vi "Test Executive.vi"(11 "Module Config":T30={"Name"="Test Executive", "Parent Q"=refnum, "Is Child?"=FALSE, "Index"=0, "Dirs"={"Root"=path "C:/MTE", "Config"=path "C:/MTE/Config", "Logs"=path "C:/MTE/Logs", "Reports"=path "C:/ATE/Reports", "App Data"=path "C:/ProgramData/Test Executive"}, "Simulate"=FALSE, "SimCtrl"=refnum}) -> ()   [LabVIEW 2018] (continued)
          frame "Simulate OFF", "Simulate ON" {
            n2666 = call <vilib>:"Menu.Simulate, Set Menu State.vi"("Menu Tag"=w5387, "Menu Ref"=w5388) -> ("Sim ON"=w5386:bool)  [unwired: 8 in, 1 out]
            n2667 = To Variant(anything=w5386) -> (Variant=w5390:variant)
            n2668 = call <vilib>:"Q.Enqueue App.vi"("Data1"=w5390, "Task Name"="Simulate", "Q In"=w5391) -> ()  [unwired: 7 in, 2 out]
          }
          frame "Show Station Module" {
            n2669 = call <vilib>:"Q.Enqueue Task.vi"("Task Name"="Station Module - Show", "Q In"=w5393) -> ()  [unwired: 8 in, 2 out]
          }
          frame "Mode Manager" {
            n2670 = call <vilib>:"Q.Enqueue Task.vi"("Task Name"="Config - Mode Manager", "Q In"=w5395) -> ()  [unwired: 8 in, 2 out]
          }
          frame "Local Station" {
            n2671 = call <vilib>:"Q.Enqueue Task.vi"("Task Name"="Config - Set Local Station Cfg", "Q In"=w5397) -> ()  [unwired: 8 in, 2 out]
          }
          frame "Test Executive" {
            n2672 = call <vilib>:"Q.Enqueue Task.vi"("Task Name"="Config - Set Test Exec Cfg", "Q In"=w5399) -> ()  [unwired: 8 in, 2 out]
          }
          frame "File Sync" {
            n2673 = To Variant(anything=TRUE) -> (Variant=w5400:variant)
            n2674 = call <vilib>:"Q.Enqueue Task.vi"("Data1"=w5400, "Task Name"="Config - Set File Sync", "Q In"=w5403) -> ()  [unwired: 7 in, 2 out]
          }
          frame "File Rotate" {
            n2675 = call <vilib>:"File.Rotate.Manager - Config Dialog.vi"("QName"="FileRotate") -> ()  [unwired: 9 in, 2 out]
          }
          frame "Test Reports" {
            n2676 = To Variant(anything=TRUE) -> (Variant=w5405:variant)
            n2677 = call <vilib>:"Q.Enqueue Task.vi"("Data1"=w5405, "Task Name"="Config - Set Reports", "Q In"=w5408) -> ()  [unwired: 7 in, 2 out]
          }
          frame "Route Check" {
            n2678 = call <vilib>:"Q.Enqueue Task.vi"("Task Name"="Route Check", "Q In"=w5410) -> ()  [unwired: 8 in, 2 out]
          }
          frame "Show PLC State" {
            n2679 = call <vilib>:"Q.Enqueue Task.vi"("Task Name"="PLC - Show State", "Q In"=w5412) -> ()  [unwired: 8 in, 2 out]
          }
          frame "Show Block Diagram" {
            n2680 = call <vilib>:"Module.Window, Q Task.vi"("Action"=Window.Task,_Action."Open Block Diagram()", "Q In"=w5414) -> ()  [unwired: 8 in, 2 out]
          }
          frame "Go to Maint Tab" {
            n2681 = call <vilib>:"Module.Window, Q Task.vi"("Show"=TRUE, "Action"=Window.Task,_Action."Go To Maint Tab()", "Q In"=w5417) -> ()  [unwired: 7 in, 2 out]
          }
        }
      }
      event "Configure Reports": Value Change {
        n2682 = event-data() -> ()  [unwired: 1 in, 6 out]
        n2683 = To Variant(anything=TRUE) -> (Variant=w5421:variant)
        n2684 = call <vilib>:"Q.Enqueue Task.vi"("Data1"=w5421, "Task Name"="Config - Set Reports", "Q In"=w5418) -> ()  [unwired: 7 in, 2 out]
      }
      event "Open SW Version File": Value Change {
        n2685 = event-data() -> ()  [unwired: 1 in, 6 out]
        n2686 = local read "SW Check Config"() -> (w5424:T12)
        n2687 = Unbundle By Name(w5424) -> ("SW Version List File"=w5423:path)
        n2688 = call <vilib>:"File.Open File or Folder.vi"("Path"=w5423) -> ("Error Out"=w5422:errorcluster)  [unwired: 10 in]
        n2689 = call <vilib>:"Clear Errors.vi"("error in (no error)"=w5422) -> ()  [unwired: 5 in, 2 out]
      }
      event "Open RprFldr": Value Change {
        n2690 = event-data() -> ()  [unwired: 1 in, 6 out]
        n2691 = for {
          tunnel: "Open RprFldr" -> [w5438] mode=indexing
          tunnel: [w5437] -> w5433
          i -> [w5437]
          stop <- w5436 stop-if-true
          n2692 = Unbundle By Name(w5438) -> ("Open"=w5436:bool)
        }
        n2693 = local read "Report Config"() -> (w5431:T17[])
        n2694 = Array Size(array=w5431) -> (size(s)=w5430:i32)
        n2695 = Index Array(array=w5431, index=w5433) -> (element=w5432:T17)
        n2696 = Unbundle By Name(w5432) -> ("Seq_Dir"=w5426:cluster{"Sequence":string, "Folder":path}[])
        n2697 = Initialize Array(cluster{"Open":bool} {"Open"=FALSE} ("Item"), w5430) -> (w5428:cluster{"Open":bool}[])
        n2698 = Index Array(array=w5426) -> (element=w5427:cluster{"Sequence":string, "Folder":path})  [unwired: 1 in]
        n2699 = local write "Open RprFldr"(w5428) -> ()
        n2700 = Unbundle By Name(w5427) -> ("Folder"=w5425:path)
        n2701 = call <vilib>:"File.Open File or Folder.vi"("Path"=w5425) -> ("Error Out"=w5435:errorcluster)  [unwired: 10 in]
        n2702 = call <vilib>:"Clear Errors.vi"("error in (no error)"=w5435) -> ()  [unwired: 5 in, 2 out]
      }
      event "Sync Now": Value Change {
        n2703 = event-data() -> ()  [unwired: 1 in, 6 out]
        n2704 = To Variant(anything=FALSE) -> (Variant=w5441:variant)
        n2705 = call <vilib>:"Q.Enqueue Task.vi"("Data1"=w5441, "Task Name"="Config - Set File Sync", "Q In"=w5440) -> ()  [unwired: 7 in, 2 out]
        "Force Sync Now" <- TRUE ("Force Sync Now")
      }
      event "Auto Scroll": Value Change {
        n2706 = event-data() -> ()  [unwired: 1 in, 6 out]
        n2707 = call <vilib>:"Q.Enqueue Task.vi"("Task Name"="Update Result Table", "Q In"=w5445) -> ()  [unwired: 8 in, 2 out]
      }
      event "LoadLimFile": Value Change {
        n2708 = event-data() -> ()  [unwired: 1 in, 6 out]
        n2709 = call <vilib>:"Q.Enqueue Task.vi"("Task Name"="Read Limits from Oper File", "Q In"=w5446) -> ()  [unwired: 8 in, 2 out]
      }
      event "PLC Enable": Value Change {
        n2710 = event-data() -> ()  [unwired: 1 in, 6 out]
        n2711 = call <vilib>:"Q.Enqueue Task.vi"("Task Name"="PLC - Enable", "Q In"=w5448) -> ()  [unwired: 8 in, 2 out]
      }
      event "Step Run": Value Change {
        n2712 = event-data() -> ()  [unwired: 1 in, 6 out]
        n2713 = property on="Inc Step" class="Bool"("DisabledEnum"=T36."Disabled and Grayed Out" ("Disabled")) -> ()  [unwired: 2 in, 2 out]
        n2714 = property on="Step Run" class="Bool"("DisabledEnum"=T36."Disabled and Grayed Out" ("Disabled")) -> ()  [unwired: 2 in, 2 out]
        n2715 = property on="Pause" class="Bool (strict)"("Value"=FALSE ("Single Step")) -> ()  [unwired: 2 in, 2 out]
      }
      event "Show Station Module": Value Change {
        n2716 = event-data() -> ()  [unwired: 1 in, 6 out]
        n2717 = call <vilib>:"Q.Enqueue Task.vi"("Task Name"="Station Module - Show", "Q In"=w5453) -> ()  [unwired: 8 in, 2 out]
      }
      event "Clear Warnings": Value Change {
        n2718 = event-data() -> ()  [unwired: 1 in, 6 out]
        n2719 = To Variant(anything=TestExec.Health_State_Command."Clear Warnings" ("Health State Cmd")) -> (Variant=w5456:variant)
        n2720 = call <vilib>:"Q.Enqueue App.vi"("Data1"=w5456, "Task Name"="Health Status", "Q In"=w5455) -> ()  [unwired: 7 in, 2 out]
      }
      event Value Change {
        n2721 = event-data() -> ()  [unwired: 1 in, 6 out]
        n2722 = call <vilib>:"Q.Enqueue App.vi"("Task Name"="Set Logging Level", "Q In"=w5460) -> ()  [unwired: 8 in, 2 out]
      }
      event "Go to Health Details": Value Change {
        n2723 = event-data() -> ()  [unwired: 1 in, 6 out]
        n2724 = local write "Health Tab"(0) -> ()
        n2725 = local write "Funct Tab"(T5."Health Status" ("Funct Tab")) -> ()
      }
      event "Status": Shortcut Menu Selection (User) {
        n2726 = event-data() -> ("ItemTag"=w5463:string)  [unwired: 1 in, 7 out]
        n2727 = case shown="\"Status_Open_in_Win\"" w5463 {
          frame "False", Default {
          }
          frame "Status_Open_in_Win" {
            n2728 = local read "Status"() -> (w5465:string)
            n2729 = call "Dialog.Launch Simple Text Info Window.vi"("Text"=w5465, "Title"="Status") -> ()  [unwired: 10 in]
          }
        }
      }
      event "Test Cycle Cnt Reset": Value Change {
        n2730 = event-data() -> ()  [unwired: 1 in, 6 out]
        n2731 = Unbundle By Name(w5468) -> ("Cfg.Dirs.Logs"=w5467:path)
        n2732 = call "TestExec.Event Counter Log.vi"("Root Name"="Test Cycle Count", "Log Folder"=w5467, "Reset"=TRUE) -> ("Event Cnt Out"=→"Total Test Cycles":i32)  [unwired: 8 in]
      }
      event "Go to Test Metric Details": Value Change {
        n2733 = event-data() -> ()  [unwired: 1 in, 6 out]
        n2734 = local write "Funct Tab"(T5."Test Reports and History" ("Funct Tab")) -> ()
      }
      event "Kill Auto Launch": Value Change {
        n2735 = event-data() -> ()  [unwired: 1 in, 6 out]
        n2736 = call <vilib>:"Q.Enqueue Task.vi"("Task Name"="Repeat Kill", "Q In"=w5473) -> ()  [unwired: 8 in, 2 out]
      }
      event Timeout {
        n2737 = event-data() -> ()  [unwired: 1 in, 3 out]
        n2738 = local read "Test Ctrl Tab"() -> (w5474:enum32{"Idle", "Running", "Completed"})
        n2739 = case shown="\"Idle\", Default" w5474 {
          frame "Idle", Default {
            # "Do Nothing"
          }
          frame "Running" {
            n2740 = local read "Start Time"() -> (w5478:timestamp)
            n2741 = Get Date/Time In Seconds() -> (seconds since 1Jan1904=w5479:timestamp)
            n2742 = local read "Progress"() -> (→"Progress 2":dbl)
            n2743 = Subtract(x=w5479, y=w5478) -> (x-y=w5475:dbl)
            n2744 = call "Time.Secs to H_M_S Duration.vi"("Total Secs"=w5475) -> ("Duration(HH:MM:SS)"=w5476:string)  [unwired: 10 in]
            n2745 = local write "Duration(s)"(w5475) -> ()
            n2746 = local write "Duration(HH:MM:SS)"(w5476) -> ()
          }
        }
      }
      event "Show Only Failures", "Filter": Value Change {
        n2747 = event-data() -> ()  [unwired: 1 in, 6 out]
        n2748 = call <vilib>:"Q.Enqueue Task.vi"("Task Name"="Update Result Table", "Q In"=w5480) -> ()  [unwired: 8 in, 2 out]
      }
      event "Clear Errors": Value Change {
        n2749 = event-data() -> ()  [unwired: 1 in, 6 out]
        n2750 = To Variant(anything=TestExec.Health_State_Command."Clear Errors" ("Health State Cmd")) -> (Variant=w5483:variant)
        n2751 = call <vilib>:"Q.Enqueue App.vi"("Data1"=w5483, "Task Name"="Health Status", "Q In"=w5482) -> ()  [unwired: 7 in, 2 out]
      }
      event "Clear Errors and Warnings": Value Change {
        n2752 = event-data() -> ()  [unwired: 1 in, 6 out]
        n2753 = To Variant(anything=TestExec.Health_State_Command."Clear All" ("Health State Cmd")) -> (Variant=w5487:variant)
        n2754 = call <vilib>:"Q.Enqueue App.vi"("Data1"=w5487, "Task Name"="Health Status", "Q In"=w5486) -> ()  [unwired: 7 in, 2 out]
      }
      event Value Change {
        n2755 = event-data() -> ()  [unwired: 1 in, 6 out]
        n2756 = call <vilib>:"Q.Enqueue Task.vi"("Task Name"="Test Metrics - Update", "Q In"=w5490) -> ()  [unwired: 8 in, 2 out]
      }
      event "Test Metrics Reset": Value Change {
        n2757 = event-data() -> ()  [unwired: 1 in, 6 out]
        n2758 = call <vilib>:"Q.Enqueue Task.vi"("Task Name"="Test Metrics - Reset", "Q In"=w5492) -> ()  [unwired: 8 in, 2 out]
      }
      event User Event {
        n2759 = event-data() -> ()  [unwired: 1 in, 5 out]
      }
      event "Start": Value Change {
        n2760 = event-data() -> ()  [unwired: 1 in, 6 out]
        n2761 = call <vilib>:"Q.Enqueue Seq.vi"("Seq Task Name"="Test Start", "Q In"=w5495) -> ()  [unwired: 8 in, 2 out]
      }
      event "SN": Value Change {
        n2762 = event-data() -> ()  [unwired: 1 in, 6 out]
        n2763 = local read "SN"() -> (w5500:string)
        n2764 = call "TestExec.Parse Barcode to PN and SN.vi"("Barcode PN SN Format"="Barcode PN SN Format", "Barcode"=w5500) -> ("PN"=→"PN":string, "SN"=w5499:string)  [unwired: 8 in]
        n2765 = local write "SN"(w5499) -> ()
        n2766 = String Length(string=w5499) -> (length=w5502:i32)
        n2767 = case shown="0..18" w5502 {
          tunnel: [u32 16 ("F2") u32 20 ("F1")] -> w5501
          frame Default {
          }
          frame 0..18 {
          }
        }
        n2768 = call <vilib>:"Q.Enqueue Task.vi"("Task Name"="Operator - SN Change", "Q In"=w5503) -> ()  [unwired: 8 in, 2 out]
        n2769 = property on="SN" class="Str"("Text.FontSize"=w5501) -> ()  [unwired: 2 in, 2 out]
      }
      event "Run Utility": Value Change {
        w5507 = "SeqCmd"
        n2770 = event-data() -> ()  [unwired: 1 in, 6 out]
        n2771 = property on="Utility INI Config File" class="Ring (strict)"() -> ("Strings []"=w5519:string[])  [unwired: 2 in, 2 out]
        n2772 = Index Array(array=w5519, index="Utility INI Config File") -> (element=w5517:string)
        n2773 = Build Array(w5517) -> (w5516:string[])
        n2774 = To Variant(anything="CreateUUTFolder") -> (Variant=w5512:variant)
        n2775 = To Variant(anything=w5516) -> (Variant=w5514:variant)
        n2776 = To Variant(anything="RunUtility") -> (Variant=w5509:variant)
        n2777 = To Variant(anything=string[] []) -> (Variant=w5508:variant)
        n2778 = call <vilib>:"Q.Enqueue Task.vi"("Data2"=w5512, "Data1"=w5508, "Task Name"=w5507, "Q In"=w5520) -> ("Q Out"=w5515:refnum<queue>)  [unwired: 6 in, 1 out]
        n2779 = call <vilib>:"Q.Enqueue Task.vi"("Data2"=w5509, "Data1"=w5514, "Task Name"=w5507, "Q In"=w5515) -> ()  [unwired: 6 in, 2 out]
      }
      event "Run Exe": Value Change {
        w5525 = "SeqCmd"
        n2780 = event-data() -> ()  [unwired: 1 in, 6 out]
        n2781 = Path To String(path="Exe Path") -> (string=w5523:string)
        n2782 = Build Array (concatenate)(w5523, "Args") -> (w5521:string[])
        n2783 = To Variant(anything="CreateUUTFolder") -> (Variant=w5530:variant)
        n2784 = To Variant(anything=w5521) -> (Variant=w5532:variant)
        n2785 = To Variant(anything="RunExe") -> (Variant=w5527:variant)
        n2786 = To Variant(anything=string[] []) -> (Variant=w5526:variant)
        n2787 = call <vilib>:"Q.Enqueue Task.vi"("Data2"=w5530, "Data1"=w5526, "Task Name"=w5525, "Q In"=w5534) -> ("Q Out"=w5533:refnum<queue>)  [unwired: 6 in, 1 out]
        n2788 = call <vilib>:"Q.Enqueue Task.vi"("Data2"=w5527, "Data1"=w5532, "Task Name"=w5525, "Q In"=w5533) -> ()  [unwired: 6 in, 2 out]
      }
      event "Zoom Left": Value Change {
        n2789 = event-data() -> ()  [unwired: 1 in, 6 out]
        n2790 = property on="Left Image" class="Pict"("ZoomFactor"="Zoom Left") -> ()  [unwired: 2 in, 2 out]
      }
      event "Zoom Img": Value Change {
        n2791 = event-data() -> ()  [unwired: 1 in, 6 out]
        n2792 = property on="OperPict" class="Pict"("ZoomFactor"="Zoom Img") -> ()  [unwired: 2 in, 2 out]
      }
      event "Zoom Right": Value Change {
        n2793 = event-data() -> ()  [unwired: 1 in, 6 out]
        n2794 = property on="Rigth Image" class="Pict"("ZoomFactor"="Zoom Right") -> ()  [unwired: 2 in, 2 out]
      }
      event "Operator": Value Change {
        n2795 = event-data() -> ()  [unwired: 1 in, 6 out]
        n2796 = call <vilib>:"Q.Enqueue Task.vi"("Task Name"="Operator - Operator Change", "Q In"=w5539) -> ()  [unwired: 8 in, 2 out]
      }
      event "Mode": Value Change {
        n2797 = event-data() -> ()  [unwired: 1 in, 6 out]
        n2798 = To Variant(anything=FALSE) -> (Variant=w5540:variant)
        n2799 = call <vilib>:"Q.Enqueue Task.vi"("Data1"=w5540, "Task Name"="Operator - Set Mode", "Q In"=w5542) -> ()  [unwired: 7 in, 2 out]
      }
      event Value Change {
        n2800 = event-data() -> ()  [unwired: 1 in, 6 out]
        n2801 = call <vilib>:"Q.Enqueue Task.vi"("Task Name"="Options - Set", "Q In"=w5544) -> ()  [unwired: 8 in, 2 out]
      }
      event "Open Event Log": Value Change {
        n2802 = event-data() -> ()  [unwired: 1 in, 6 out]
        n2803 = call <vilib>:"Event Log.Show.vi"() -> ()  [unwired: 11 in, 1 out]
      }
      event "Abort": Value Change {
        n2804 = event-data() -> ()  [unwired: 1 in, 6 out]
        n2805 = call <vilib>:"Q.Enqueue Seq.vi"("Top of Q"=TRUE, "Seq Task Name"="Test Abort", "Q In"=w5546) -> ()  [unwired: 7 in, 2 out]
        n2806 = for {
          N: 5 -> [_]
          n2807 = call "Abort.Send Abort or Done Notificaiton.vi"("Abort(T)/Done(F)"=TRUE) -> ()  [unwired: 10 in, 1 out]
          n2808 = Wait (ms)(milliseconds to wait=u32 10) -> ()  [unwired: 1 out]
        }
        "Abort Flag" <- TRUE ("Abort Flag")
      }
      event "Set TE Sta Cfg": Value Change {
        n2809 = event-data() -> ()  [unwired: 1 in, 6 out]
        n2810 = call <vilib>:"Q.Enqueue Task.vi"("Task Name"="Config - Set Test Exec Cfg", "Q In"=w5554) -> ()  [unwired: 8 in, 2 out]
      }
      event "Sim Wiggler Start": Value Change {
        n2811 = event-data() -> ()  [unwired: 1 in, 6 out]
        n2812 = call <vilib>:"Q.Enqueue Task.vi"("Task Name"="PLC - Set Start", "Q In"=w5555) -> ()  [unwired: 8 in, 2 out]
      }
      event "Test Reset": Value Change {
        n2813 = event-data() -> ()  [unwired: 1 in, 6 out]
        n2814 = call <vilib>:"Q.Enqueue Seq.vi"("Seq Task Name"="Test Reset" ("Task Name"), "Q In"=w5558) -> ()  [unwired: 8 in, 2 out]
      }
      event Value Change {
        n2815 = event-data() -> ()  [unwired: 1 in, 6 out]
        n2816 = call <vilib>:"Q.Enqueue Task.vi"("Task Name"="Operator - Set Result EN", "Q In"=w5560) -> ()  [unwired: 8 in, 2 out]
      }
      event "Exit Sta module": Value Change {
        n2817 = event-data() -> ()  [unwired: 1 in, 6 out]
        n2818 = local read "StaModule"() -> (w5561:string)
        n2819 = call <vilib>:"Q.Enqueue Exit.vi"("Q Name"=w5561) -> ()  [unwired: 9 in, 2 out]
      }
      event "Open Image File": Value Change {
        n2820 = event-data() -> ()  [unwired: 1 in, 6 out]
        n2821 = local read "Image Path"() -> (w5563:path)
        n2822 = call <vilib>:"File.Open File or Folder.vi"("Path"=w5563) -> ("Error Out"=w5562:errorcluster)  [unwired: 10 in]
        n2823 = call <vilib>:"Clear Errors.vi"("error in (no error)"=w5562) -> ()  [unwired: 5 in, 2 out]
      }
      event "Create RTF Report": Value Change {
        n2824 = event-data() -> ()  [unwired: 1 in, 6 out]
        n2825 = call <vilib>:"Q.Enqueue Task.vi"("Task Name"="Result - RTF Report", "Q In"=w5565) -> ()  [unwired: 8 in, 2 out]
      }
      event "Open Root Folder": Value Change {
        n2826 = event-data() -> ()  [unwired: 1 in, 6 out]
        n2827 = Unbundle By Name(w5567) -> ("Cfg.Dirs.Root"=w5566:path)
        n2828 = call <vilib>:"File.Open File or Folder.vi"("Path"=w5566) -> ("Error Out"=w5568:errorcluster)  [unwired: 10 in]
        n2829 = call <vilib>:"Clear Errors.vi"("error in (no error)"=w5568) -> ()  [unwired: 5 in, 2 out]
      }
      event "Test Status Tab": Value Change {
        n2830 = event-data() -> ("NewVal"=w5569:T6)  [unwired: 1 in, 5 out]
        n2831 = local write "Test Status Tab Sel"(w5569) -> ()
      }
      event "Test Status Tab Sel": Value Change {
        n2832 = event-data() -> ()  [unwired: 1 in, 6 out]
        n2833 = local write "Test Status Tab"("Test Status Tab Sel") -> ()
      }
    }
  }
  n2834 = Build Path(base path=w3, name or relative path="Data\\ArchiveTemp") -> (appended path=w1:path)
  n2835 = call "PLC.Check Enabled State.vi"("Config Folder"=w28) -> ("error out"=w18:errorcluster, "Type"=w11:T86, "Enabled"=w19:bool)  [unwired: 8 in]
  n2836 = call <vilib>:"File.Rotate.Manager - Core.vi"("Q Name"="FileRotate", "Config Folder"=w6) -> ()  [unwired: 10 in]
  n2837 = call "File.Archive Dir Mover.vi"("TempLocal"=w1, "Parent Q"=w8, "Q Name"="ArchiveMover") -> ()  [unwired: 9 in]
  n2838 = control-ref of="Wiggler"() -> (w12:refnum<vi>)
  n2839 = property on="Wiggler" class="Bool (strict)"("Visible"=TRUE) -> ()  [unwired: 2 in, 2 out]
  n2840 = case shown="True" w19 {
    tunnel: w4 -> [w5575 w5582]
    tunnel: [w5572 _] -> _
    tunnel: w18 -> [_ _]
    tunnel: w11 -> [_ w5577]
    frame False {
      w5571 = "PLC" ("menu tag")
      w5576 = FALSE ("Visible")
      n2841 = Unbundle By Name(w5575) -> ("Menu Ref"=w5573:refnum<k9>)
      n2842 = property on="PLC" class="Bool (strict)"("Visible"=w5576) -> ()  [unwired: 2 in, 2 out]
      n2843 = property on="PLC Enable" class="Bool (strict)"("Visible"=w5576) -> ()  [unwired: 2 in, 2 out]
      n2844 = Set Menu Item Info(7:w5571, 9:FALSE ("enabled"), 10:w5571, 11:w5573) -> (0:w5572:errorcluster)  [unwired: 3 in, 1 out]
    }
    frame True {
      n2845 = Unbundle By Name(w5582) -> ("Main Q"=w5581:refnum<queue>, "Cfg.Dirs.Config"=w5580:path)
      n2846 = control-ref of="PLC"() -> (w5584:refnum<vi>)
      n2847 = property on="PLC Enable" class="Bool (strict)"("Visible"=TRUE) -> ()  [unwired: 2 in, 2 out]
      n2848 = case shown="\"Dial 800\"" w5577 {
        tunnel: w5584 -> [_ w5591 w5596]
        tunnel: "PLC" ("Q Name") -> [_ w5590 w5595]
        tunnel: w5581 -> [_ w5589 w5594]
        tunnel: w5580 -> [_ w5588 w5593]
        tunnel: TRUE -> [_ w5587 w5592]
        frame "None", Default {
        }
        frame "Dial 750" {
          n2849 = call "PLC.Dial750.vi"("PLC Indicator"=w5591, "Is Child"=w5587, "Config Dir"=w5588, "Name"=w5590, "TE Q"=w5589) -> ()  [unwired: 7 in]
        }
        frame "Dial 800" {
          n2850 = call "PLC.Dial800.vi"("PLC Indicator"=w5596, "Is Child"=w5592, "Config Dir"=w5593, "Name"=w5595, "TE Q"=w5594) -> ()  [unwired: 7 in]
        }
      }
      n2851 = property on="PLC" class="Bool (strict)"("Visible"=TRUE) -> ()  [unwired: 2 in, 2 out]
      "PLC" <- FALSE ("PLC")
    }
  }
  n2852 = call "CircleTest.Wiggler Manager.vi"("Wiggler LED Ref"=w12, "ConfigDir"=w13, "ParentQ"=w14, "Q Name"="Wiggler") -> ()  [unwired: 8 in]
  "Wiggler" <- FALSE ("Wiggler")
